vi "Clear Event Registration.vi"(8 "error in (no error)":errorcluster, 11 "Worker in":refnum<class "Worker.lvclass">) -> (0 "error out":errorcluster, 3 "Worker out":refnum<class "Worker.lvclass">)   [LabVIEW 2023, in "Worker.lvlib" / "Worker.lvclass"]
doc: "Clean up all User Event registrations used by the parent Worker UI."
uses:
  Worker.lvclass
  Worker.lvclass/Worker.ctl
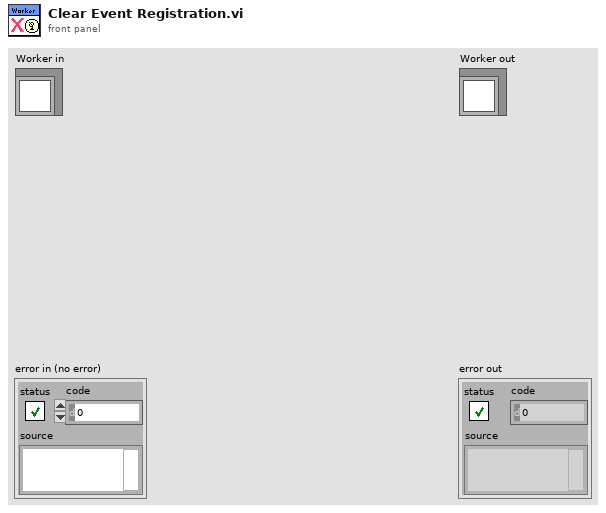
[diagram p1: front panel]
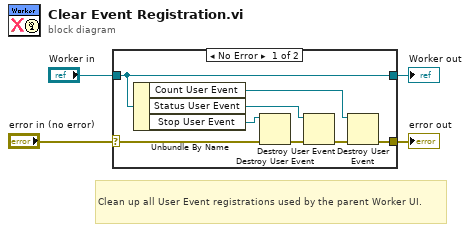
[diagram p0: block diagram]
diagram:
  # "Clean up all User Event registrations used by the parent Worker UI."
  n1 = case shown="No Error" "error in (no error)" {
    selector: "error in (no error)" -> [w6 w14]
    tunnel: [w5 w14] -> w3
    tunnel: [w7 w13] -> w1
    tunnel: "Worker in" -> [w7 w13]
    frame No Error {
      n2 = Unbundle By Name(w7) -> ("Count User Event"=w8:refnum<user-event>, "Status User Event"=w10:refnum<user-event>, "Stop User Event"=w12:refnum<user-event>)
      n3 = Destroy User Event(user event=w12, error in=w6) -> (error out=w11:errorcluster)
      n4 = Destroy User Event(user event=w10, error in=w11) -> (error out=w9:errorcluster)
      n5 = Destroy User Event(user event=w8, error in=w9) -> (error out=w5:errorcluster)
    }
    frame Error {
    }
  }
  "error out" <- w3
  "Worker out" <- w1
